vi "SVX Buffer Waterfall Graph (Single Plot).vi"(5 "reset on change to dx (F)":bool, 6 "number of spectra (40)":i32=40, 7 "reset? (F)":bool, 8 "error in (no error)":errorcluster, 9 "dz":dbl=1.0, 10 "initial z0":dbl, 11 "plot":cluster{"x0":dbl, "dx":dbl, "Y":dbl[]}) -> (0 "error out":errorcluster, 3 "waterfall graph data out":T2={"z0"=0.0, "dz"=1.0, "plots"=[]})   [LabVIEW 2017, in "SoundVib_SpectralDisplay.lvlib"]
doc: "Buffers signals and returns the buffered signals up to a maximum count. If you use this VI with the Waterfall Graph, the display mimics the behavior of a chart. Wire data to the <B>waterfall graph data</B> input to determine the polymorphic instance to use or manually select the instance."
uses:
  <vilib>/addons/Sound and Vibration/Order Analysis/Data Presentation/SoundVib_SpectralDisplay.lvlib
panel:
  in  "waterfall graph data":T1={"z0"=0.0, "dz"=1.0, "Plots"=[]}
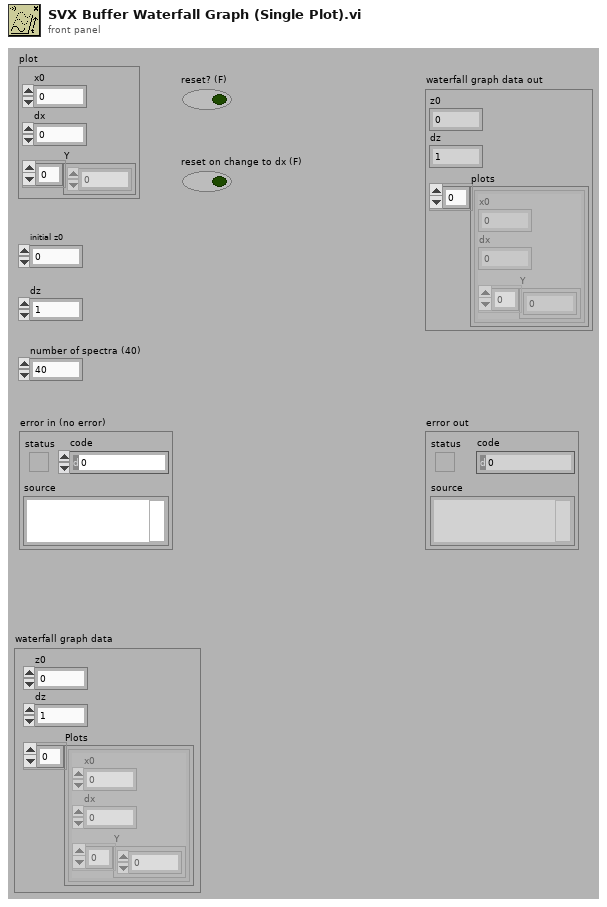
[diagram p1: front panel]
types:
  T1 = cluster{"z0":dbl, "dz":dbl, "Plots":cluster{"x0":dbl, "dx":dbl, "Y":dbl[]}[]}
  T2 = cluster{"z0":dbl, "dz":dbl, "plots":cluster{"x0":dbl, "dx":dbl, "Y":dbl[]}[]}
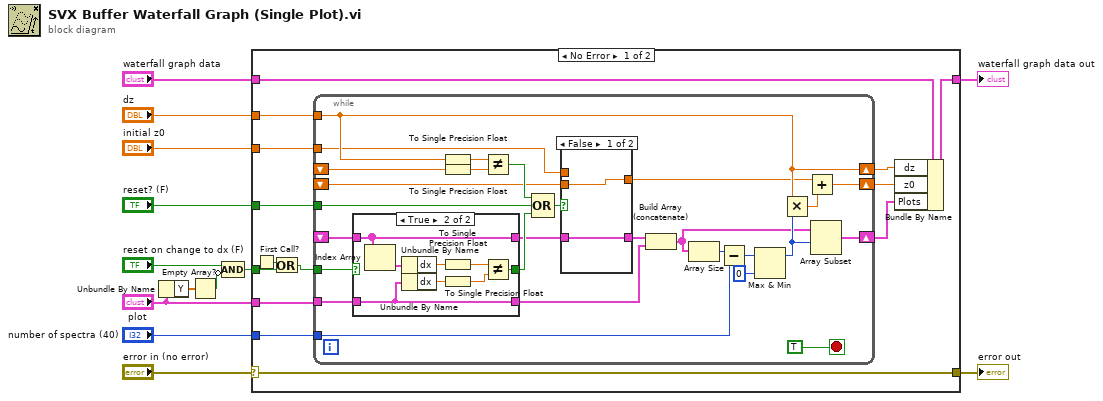
[diagram p0: block diagram]
diagram:
  n1 = Unbundle By Name("plot") -> ("Y"=w4:dbl[])
  n2 = Empty Array?(array=w4) -> (empty?=w3:bool)
  n3 = Compound Arithmetic op=AND("reset on change to dx (F)", invert w3) -> (w1:bool)
  n4 = case shown="No Error" "error in (no error)" {
    selector: "error in (no error)" -> [w27 w70]
    tunnel: [w27 w70] -> w12
    tunnel: "reset? (F)" -> [w21 _]
    tunnel: "number of spectra (40)" -> [w26 _]
    tunnel: "plot" -> [w20 _]
    tunnel: [w16 w69] -> w9
    tunnel: "dz" -> [w24 _]
    tunnel: "initial z0" -> [w23 _]
    tunnel: "waterfall graph data" -> [w22 w69]
    tunnel: w1 -> [w19 _]
    frame No Error {
      n5 = First Call?() -> (First Call?: T/F=w14:bool)
      n6 = Or(x=w14, y=w19) -> (x .or. y?=w15:bool)
      n7 = while {
        tunnel: w26 -> [w47]
        shift-right: [w52] -> w25
        shift-left: _ -> [w35]
        tunnel: w21 -> [w43]
        shift-right: [w48] -> w18
        shift-left: _ -> [w36]
        tunnel: w20 -> [w34]
        tunnel: w24 -> [w44]
        tunnel: w23 -> [w38]
        shift-right: [w44] -> w17
        shift-left: _ -> [w45]
        tunnel: w15 -> [w32]
        stop <- TRUE stop-if-true
        n8 = case shown="True" w32 {
          selector: w32 -> [w55 _]
          tunnel: w35 -> [w57 w62]
          tunnel: w34 -> [w56 w60]
          tunnel: [w55 w63] -> w33
          tunnel: [w57 w62] -> w31
          tunnel: [w56 w60] -> w30
          frame False {
          }
          frame True {
            n9 = Index Array(array=w62) -> (element=w65:cluster{"x0":dbl, "dx":dbl, "Y":dbl[]})  [unwired: 1 in]
            n10 = Unbundle By Name(w65) -> ("dx"=w64:dbl)
            n11 = Unbundle By Name(w60) -> ("dx"=w61:dbl)
            n12 = To Single Precision Float(number=w64) -> (single precision float=w59:sgl)
            n13 = To Single Precision Float(number=w61) -> (single precision float=w58:sgl)
            n14 = Not Equal?(x=w59, y=w58) -> (x != y?=w63:bool)
          }
        }
        n15 = To Single Precision Float(number=w44) -> (single precision float=w29:sgl)
        n16 = To Single Precision Float(number=w45) -> (single precision float=w28:sgl)
        n17 = Not Equal?(x=w29, y=w28) -> (x != y?=w42:bool)
        n18 = Compound Arithmetic op=OR(w42, w43, w33) -> (w41:bool)
        n19 = case shown="False" w41 {
          tunnel: w31 -> [w67 _]
          tunnel: [w67 _] -> w39
          tunnel: w38 -> [_ w68]
          tunnel: [w66 w68] -> w37
          tunnel: w36 -> [w66 _]
          frame False {
          }
          frame True {
          }
        }
        n20 = Build Array (concatenate)(w39, w30) -> (w40:cluster{"x0":dbl, "dx":dbl, "Y":dbl[]}[])
        n21 = Array Size(array=w40) -> (size(s)=w53:i32)
        n22 = Subtract(x=w53, y=w47) -> (x-y=w51:i32)
        n23 = Max & Min(x=w51, y=0) -> (max(x,y)=w46:i32)  [unwired: 1 out]
        n24 = Multiply(x=w44, y=w46) -> (x*y=w49:dbl)
        n25 = Add(x=w37, y=w49) -> (x+y=w48:dbl)
        n26 = Array Subset(array=w40, index=w46) -> (w52:cluster{"x0":dbl, "dx":dbl, "Y":dbl[]}[])  [unwired: 1 in]
      }
      n27 = Bundle By Name(cluster=w22, "dz"=w17, "z0"=w18, "Plots"=w25) -> (w16:T1)
    }
    frame Error {
    }
  }
  "waterfall graph data out" <- w9
  "error out" <- w12
